vi "PH_4_Pos_Selector.get current Axes Positions.vi"(0 "VI in":refnum<vi>, 5 "error in (no error)":errorcluster) -> (14 "VI out":refnum<vi>, 16 "Current Axes Positions":T1, 17 "No Info, Failure oder Alarm?":bool, 18 "Moving?":bool, 19 "error out":errorcluster)   [LabVIEW 2014, in "PH_4_Pos_Selector.lvlib"]
uses:
  PH_4_Pos_Selector.lvlib
  PH_4_Pos_Selector.Position.ctl
  PH_Basics/PH_AxisGUI_BaseClass/PH_AxisGUI_BaseClass.lvlib
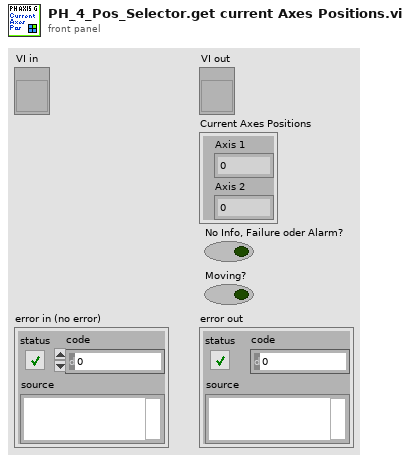
[diagram p1: front panel]
types:
  T1 = typedef "PH_4_Pos_Selector.lvlib/PH_4_Pos_Selector.Position.ctl" = cluster{"Axis 1":dbl, "Axis 2":dbl}
  T2 = typedef "PH_AxisGUI_BaseClass.lvlib/PH_AxisGUI_BaseClass.i attribute.ctl" = cluster{"Axes":T3[]}
  T3 = typedef "PH_AxisGUI_BaseClass.lvlib/PH_AxisGUI_BaseClass.Axis Attributes.ctl" = cluster{"Axis GUI Refs":T4, "Address":T5, "Name":string, "Label \"Back\"":string, "Labell \"Forth\"":string, "Moving?":bool}
  T4 = typedef "PH_AxisGUI_BaseClass.lvlib/PH_AxisGUI_BaseClass.Axis GUI Refs.ctl" = cluster{"Back":refnum<vi>, "Forth":refnum<vi>, "Status":refnum<vi>, "Target":refnum<vi>, "Address":refnum<vi>, "Status Bar":refnum<vi>, "Settings":refnum<vi>, "Activity":refnum<vi>, "Clear Error":refnum<vi>}
  T5 = typedef "PH_Stepmotor_BaseClass.lvlib/PH_Stepmotor_BaseClass.Axis Address.ctl" = cluster{"Instance":string, "Motor Nr":i32}
  T6 = typedef "PH_Stepmotor_BaseClass.lvlib/PH_Stepmotor_BaseClass.Axis Activity.ctl" = enum16{"No Information", "stopped", "running", "Failure", "Alarm", "stopped at backward ES", "stopped at foreward ES"}
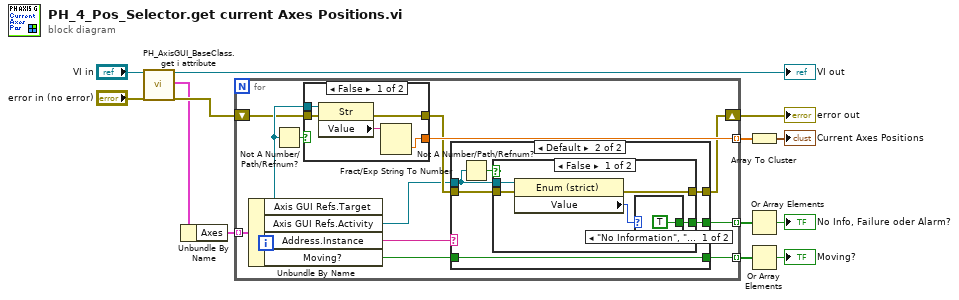
[diagram p0: block diagram]
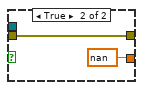
[diagram p2: hidden frame]
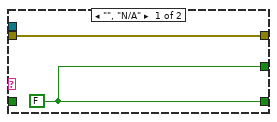
[diagram p3: hidden frame]
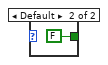
[diagram p4: hidden frame]
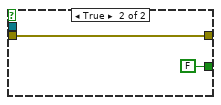
[diagram p5: hidden frame]
diagram:
  n1 = call "PH_AxisGUI_BaseClass.get i attribute.vi"("i ref in"="VI in", "error in (no error)"="error in (no error)") -> ("i ref out"=→"VI out":refnum<vi>, "i attribute"=w1:T2, "error out"=w7:errorcluster)  [unwired: 15 in]
  n2 = Unbundle By Name(w1) -> ("Axes"=w4:T3[])
  n3 = for {
    tunnel: [w25] -> w2 mode=indexing
    tunnel: w4 -> [w24] mode=indexing
    shift-right: [w16] -> w11
    shift-left: w7 -> [w19]
    tunnel: [w22] -> w8 mode=indexing
    tunnel: [w15] -> w12 mode=indexing
    n4 = Unbundle By Name(w24) -> ("Axis GUI Refs.Target"=w20:refnum<vi>, "Axis GUI Refs.Activity"=w17:refnum<vi>, "Address.Instance"=w14:string, "Moving?"=w23:bool)
    n5 = Not A Number/Path/Refnum?(number/path/refnum=w20) -> (NaN/Path/Refnum?=w21:bool)
    n6 = case shown="False" w21 {
      tunnel: w20 -> [w30 _]
      tunnel: w19 -> [w29 w32]
      tunnel: [w28 w32] -> w18
      tunnel: [w26 nan] -> w22
      frame False {
        n7 = property class="Str"(reference=w30, error in=w29) -> (error out=w28:errorcluster, "Value"=w27:string)  [unwired: 1 out]
        n8 = Fract/Exp String To Number(string=w27) -> (number=w26:dbl)  [unwired: 3 in, 1 out]
      }
      frame True {
      }
    }
    n9 = case shown="Default" w14 {
      tunnel: [w33 w40] -> w25
      tunnel: w23 -> [_ w40]
      tunnel: w18 -> [w34 w38]
      tunnel: w17 -> [_ w37]
      tunnel: [w34 w36] -> w16
      tunnel: [w33 w35] -> w15
      frame "", "N/A" {
        w33 = FALSE
      }
      frame Default {
        n10 = Not A Number/Path/Refnum?(number/path/refnum=w37) -> (NaN/Path/Refnum?=w39:bool)
        n11 = case shown="False" w39 {
          tunnel: w37 -> [w45 _]
          tunnel: w38 -> [w44 w49]
          tunnel: [w43 w49] -> w36
          tunnel: [w41 FALSE] -> w35
          frame False {
            n12 = property class="Enum (strict)"(reference=w45, error in=w44) -> (error out=w43:errorcluster, "Value"=w42:T6)  [unwired: 1 out]
            n13 = case shown="\"No Information\", \"Failure\", \"Alarm\"" w42 {
              tunnel: [TRUE FALSE] -> w41
              frame "No Information", "Failure", "Alarm" {
              }
              frame Default {
              }
            }
          }
          frame True {
          }
        }
      }
    }
  }
  "error out" <- w11
  n14 = Array To Cluster(array=w8) -> (cluster=→"Current Axes Positions":cluster{"[0]":dbl, "[1]":dbl})
  n15 = Or Array Elements(Boolean array=w12) -> (logical OR=→"No Info, Failure oder Alarm?":bool)
  n16 = Or Array Elements(Boolean array=w2) -> (logical OR=→"Moving?":bool)
